vi "Server_Init.vi"(8 "error in (no error)":errorcluster, 9 "Static Data Folder":path, 10 "API Queue":refnum<queue>, 11 "reference in":refnum<class "Server.lvclass"> caption="This control should only be used when\na sub class is inheriting this class") -> (0 "error out":errorcluster, 3 "reference out":refnum<class "Server.lvclass"> caption="This indicator should only be used when\na sub class is inheriting this class")   [LabVIEW 2023, in "Server.lvclass"]
uses:
  Server.lvclass
  API Message/API Message.lvclass
  Server.lvclass/Server.ctl
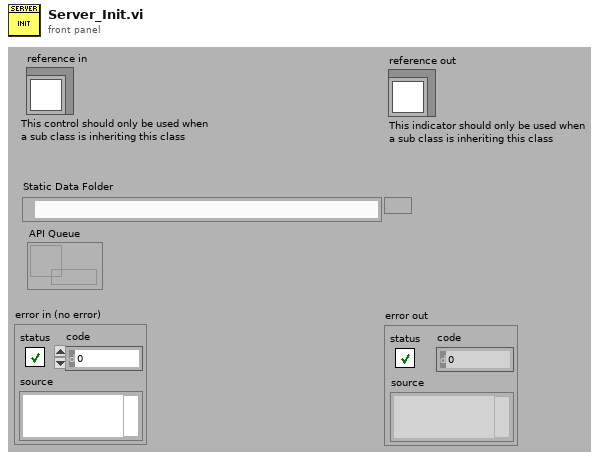
[diagram p1: front panel]
types:
  T1 = typedef "Server.lvclass/ObjectAttributes.ctl" = cluster{"Static Data":path, "MIME Types":variant, "Shutdown":bool, "API Queue":refnum<queue>}
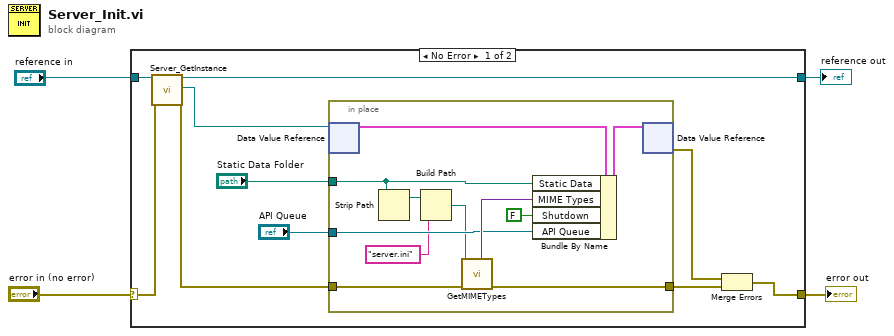
[diagram p0: block diagram]
diagram:
  n1 = case shown="No Error" "error in (no error)" {
    selector: "error in (no error)" -> [w12 w27]
    tunnel: [w13 w27] -> w3
    tunnel: "reference in" -> [w11 w26]
    tunnel: [w10 w26] -> w1
    frame No Error {
      n2 = call "Server_GetInstance.vi"("reference in"=w11, "error in (no error)"=w12) -> ("reference out"=w10:refnum<class "Server.lvclass">, "DVRRefOut"=w9:refnum<data-value>, "error out"=w8:errorcluster)  [unwired: 13 in, 2 out]
      n3 = in-place {
        in-place-border: w8 -> [w23]
        in-place-border: [w22] -> w7
        in-place-border: "Static Data Folder" -> [w15]
        in-place-border: "API Queue" -> [w19]
        n4 = in-place-dvr #1(w9) -> (w24:T1)  [unwired: 1 out]
        n5 = Strip Path(path=w15) -> (stripped path=w16:path)  [unwired: 1 out]
        n6 = Build Path(base path=w16, name or relative path="server.ini") -> (appended path=w18:path)
        n7 = call "GetMIMETypes.vi"("error in (no error)"=w23, "Config File"=w18) -> ("error out"=w22:errorcluster, "MIME Types"=w21:variant)  [unwired: 8 in]
        n8 = Bundle By Name(cluster=w24, "Static Data"=w15, "MIME Types"=w21, "Shutdown"=FALSE, "API Queue"=w19) -> (w25:T1)
        n9 = in-place-dvr #1(w25) -> (w14:errorcluster)  [unwired: 1 out]
      }
      n10 = Merge Errors(w14, w7) -> (w13:errorcluster)
    }
    frame Error {
    }
  }
  "error out" <- w3
  "reference out" <- w1
